vi "ArrayTo1DGen.vi"   [LabVIEW 2019]
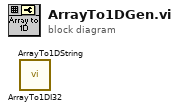
[diagram p0: block diagram]
diagram:
  n1 = call <userlib>:"ArrayTo1DI32.vi"() -> ()  [unwired: 9 in, 3 out]
  n2 = call <userlib>:"ArrayTo1DString.vi"() -> ()  [unwired: 9 in, 3 out]
